vi "forceOutputState.vi"(8 "error in (no error)":errorcluster, 9 "calibratedValues":dbl[](array[numeric]), 10 "channel_addresses":string[](array[string]), 11 "K2602 in":refnum<class "K2602.lvclass">) -> (0 "error out":errorcluster, 3 "K2602 out":refnum<class "K2602.lvclass">)   [LabVIEW 2009, in "Hardware.lvlib" / "Channels.lvlib" / "K2602.lvclass"]
uses:
  K2602.lvclass
  K2602.lvclass/K2602.ctl
  <instrlib>/Keithley 2600 Series/Keithley 2600 Series.lvlib
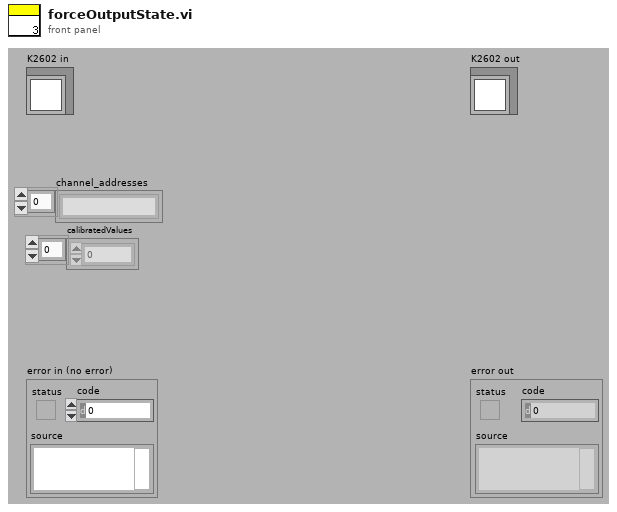
[diagram p1: front panel]
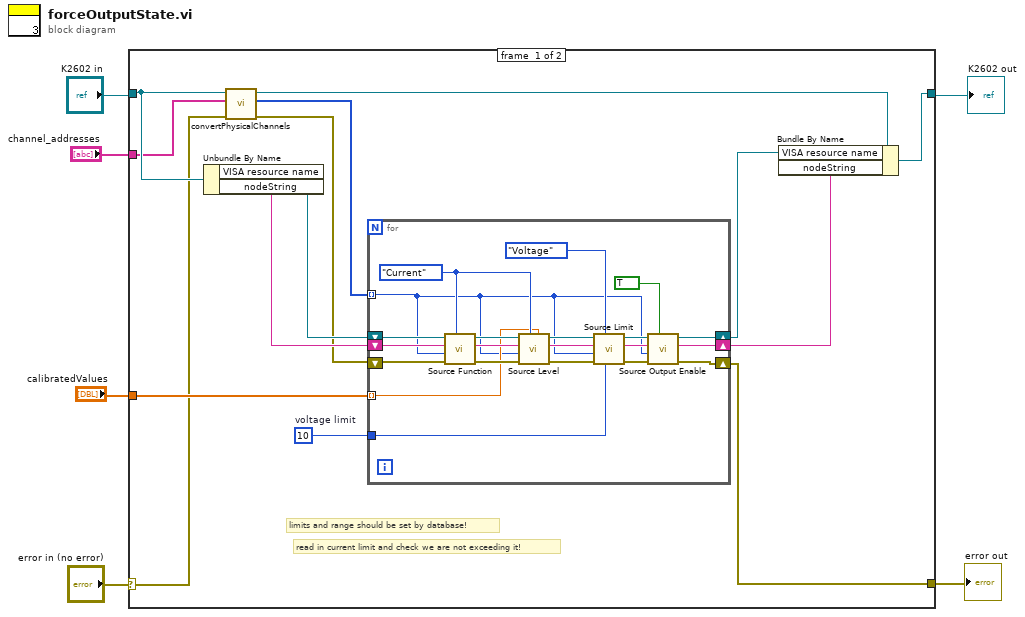
[diagram p0: block diagram]
diagram:
  n1 = case shown="No Error" "error in (no error)" {
    selector: "error in (no error)" -> [w7 w42]
    tunnel: [w12 w43] -> w2
    tunnel: "K2602 in" -> [w10 w43]
    tunnel: [w11 w42] -> w1
    tunnel: "calibratedValues" -> [w9 _]
    tunnel: "channel_addresses" -> [w8 _]
    frame #0 {
      w16 = 10  # voltage limit
      # "read in current limit and check we are not exceeding it!"
      # "limits and range should be set by database!"
      n2 = Unbundle By Name(w10) -> ("VISA resource name"=w20:refnum<visa-resource-name>, "nodeString"=w19:string)
      n3 = call "convertPhysicalChannels.vi"("error in (no error)"=w7, "physicalChannels"=w8, "K2602 in"=w10) -> ("error out"=w18:errorcluster, "channel"=w17:i32[], "K2602 out"=w15:refnum<class "K2602.lvclass">)  [unwired: 6 in]
      n4 = for {
        tunnel: w17 -> [w26] mode=indexing
        tunnel: w16 -> [w31]
        tunnel: w9 -> [w30] mode=indexing
        shift-right: [w22] -> w14
        shift-left: w20 -> [w35]
        shift-right: [w23] -> w13
        shift-left: w19 -> [w34]
        shift-right: [w24] -> w11
        shift-left: w18 -> [w33]
        w36 = enum32{"Current", "Voltage"}."Current" ("Source Function (Current)")
        n5 = call <instrlib>:"Source Function.vi"("Function (Current)"=w36, "error in (no error)"=w33, "Channel (Channel A)"=w26, "Node In"=w34, "VISA resource name"=w35) -> ("error out"=w39:errorcluster, "Node Out"=w41:string, "VISA resource name out"=w40:refnum<visa-resource-name>)  [unwired: 4 out]
        n6 = call <instrlib>:"Source Level.vi"("Level (0.000)"=w30, "Function (Current)"=w36, "error in (no error)"=w39, "Channel (Channel A)"=w26, "Node In"=w41, "VISA resource name"=w40) -> ("error out"=w29:errorcluster, "Node Out"=w37:string, "VISA resource name out"=w38:refnum<visa-resource-name>)  [unwired: 3 out]
        n7 = call <instrlib>:"Source Limit.vi"("Limit (0.000)"=w31, "Function (Current)"=enum32{"Current", "Voltage"}."Voltage" ("x"), "error in (no error)"=w29, "Channel (Channel A)"=w26, "Node In"=w37, "VISA resource name"=w38) -> ("error out"=w25:errorcluster, "Node Out"=w27:string, "VISA resource name out"=w28:refnum<visa-resource-name>)  [unwired: 3 out]
        n8 = call <instrlib>:"Source Output Enable.vi"("Output (Off)"=TRUE, "error in (no error)"=w25, "Channel (Channel A)"=w26, "Node In"=w27, "VISA resource name"=w28) -> ("error out"=w24:errorcluster, "Node Out"=w23:string, "VISA resource name out"=w22:refnum<visa-resource-name>)  [unwired: 3 in, 1 out]
      }
      n9 = Bundle By Name(cluster=w15, "VISA resource name"=w14, "nodeString"=w13) -> (w12:refnum<class "K2602.lvclass">)
    }
    frame #1 {
    }
  }
  "error out" <- w1
  "K2602 out" <- w2
